vi "RunVI.vi"   [LabVIEW 2019, in "LabJSON.lvlib"]
uses:
  LabJSON.lvlib
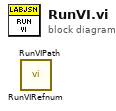
[diagram p0: block diagram]
diagram:
  n1 = call "RunVIRefnum.vi"() -> ()  [unwired: 9 in, 3 out]
  n2 = call "RunVIPath.vi"() -> ()  [unwired: 10 in, 2 out]
